vi "Get Generation Info From Proto.vi"(8 "error in":errorcluster, 10 "proto file name":string="data_store_service.proto", 11 "source proto directory":path=path "C:/dev/ASW/Source/Protos") -> (0 "error out":errorcluster, 3 "generation data":T1)   [LabVIEW 2024, in "gRPC Client Generation.lvlib"]
uses:
  gRPC Client Generation.lvlib
  Generation Data.ctl
  <vilib>/Utility/error.llb/Error Cluster From Error Code.vi
  <vilib>/ErrorRing/Error Ring.xnode
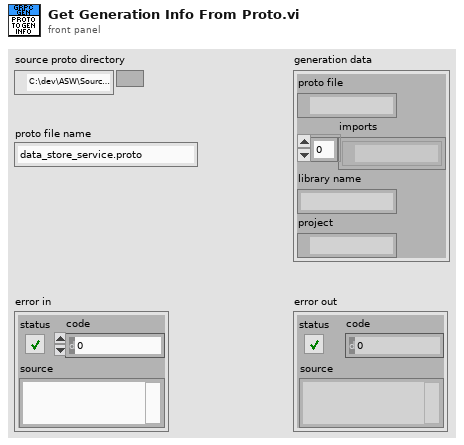
[diagram p1: front panel]
types:
  T1 = typedef "gRPC Client Generation.lvlib/Generation Data.ctl" = cluster{"proto file":path, "imports":path[], "library name":string, "project":path}
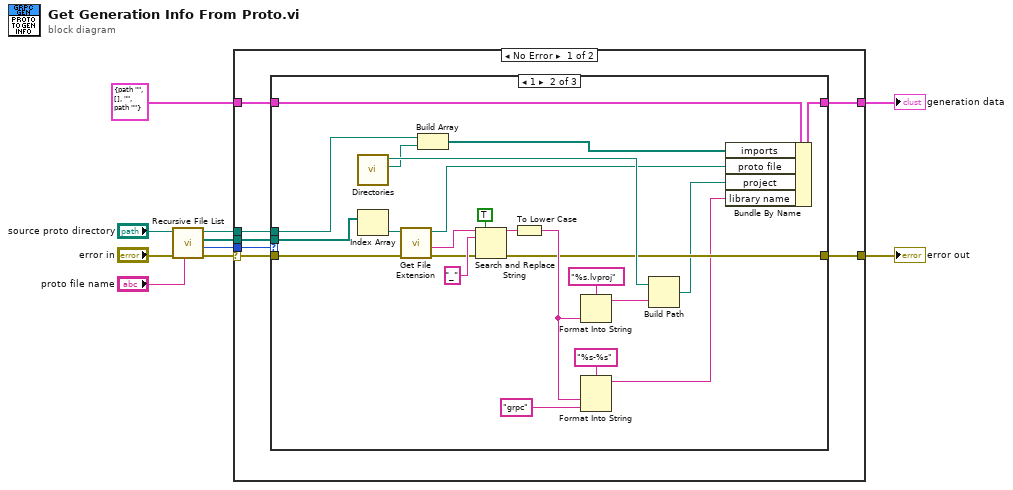
[diagram p0: block diagram]
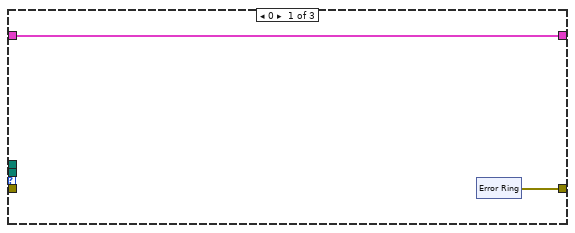
[diagram p2: hidden frame]
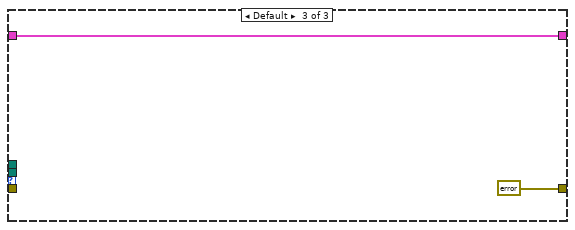
[diagram p3: hidden frame]
diagram:
  n1 = call <vilib>:"Recursive File List.vi"("pattern"="proto file name", "error in (no error)"="error in", "Folder Path"="source proto directory") -> ("error out"=w4:errorcluster, "Number of Files"=w9:i32, "All Files in Dir"=w7:path[], "dup Folder Path"=w8:path)  [unwired: 4 in, 1 out]
  n2 = case shown="No Error" w4 {
    selector: w4 -> [w14 w49]
    tunnel: w9 -> [w17 _]
    tunnel: w8 -> [w16 _]
    tunnel: w7 -> [w15 _]
    tunnel: [w13 w49] -> w3
    tunnel: T1 {"proto file"=path "", "imports"=[], "library name"="", "project"=path ""} ("generation data") -> [w12 _]
    tunnel: [w11 _] -> w1
    frame No Error {
      n3 = case shown="1" w17 {
        tunnel: w16 -> [_ w38 _]
        tunnel: w15 -> [_ w45 _]
        tunnel: w14 -> [_ w40 _]
        tunnel: [w19 w31 errorcluster {"status"=TRUE, "code"=5001, "source"="Found multiple proto files with provided name."} ("error constant")] -> w13
        tunnel: w12 -> [w18 w30 w47]
        tunnel: [w18 w24 w47] -> w11
        frame 0 {
          n4 = xnode "Error Ring"() -> ("error out"=w19:errorcluster)
        }
        frame 1 {
          n5 = call "Directories.vi"() -> ("imports"=w32:path, "src"=w33:path)  [unwired: 10 in]
          n6 = Index Array(array=w45) -> (element=w29:path)  [unwired: 1 in]
          n7 = call <vilib>:"Get File Extension.vi"("error in (no error)"=w40, "file"=w29) -> ("error out"=w39:errorcluster, "filename without extension"=w44:string, "dup file"=w25:path)  [unwired: 5 in, 2 out]
          n8 = Build Array(w38, w32) -> (w28:path[])
          n9 = Search and Replace String(replace all?=TRUE ("replace all? (F)"), input string=w44, search string="_", error in=w39) -> (result string=w43:string, error out=w31:errorcluster)  [unwired: 4 in, 2 out]
          n10 = To Lower Case(string=w43) -> (all lower case string=w35:string)
          n11 = Format Into String(format string="%s.lvproj", w35) -> (resulting string=w36:string)  [unwired: 2 in, 1 out]
          n12 = Format Into String(format string="%s-%s", w35, "grpc" ("input 1")) -> (resulting string=w26:string)  [unwired: 2 in, 1 out]
          n13 = Build Path(base path=w33, name or relative path=w36) -> (appended path=w27:path)
          n14 = Bundle By Name(cluster=w30, "imports"=w28, "proto file"=w25, "project"=w27, "library name"=w26) -> (w24:T1)
        }
        frame Default {
        }
      }
    }
    frame Error {
    }
  }
  "error out" <- w3
  "generation data" <- w1
